vi "Release Queue.vi"(8 "error in (no error)":errorcluster, 11 "Bounded Priority Queue":refnum<class "Bounded Priority Queue.lvclass">) -> (0 "error out":errorcluster, 2 "Remaining Elements":T1[](array[typedef]))   [LabVIEW 2011, in "Bounded Priority Queue.lvclass"]
uses:
  Bounded Priority Queue.lvclass
  Data.ctl
  Bounded Priority Queue.lvclass/Bounded Priority Queue.ctl
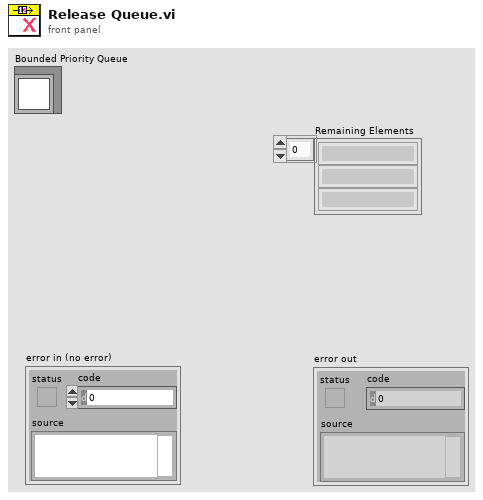
[diagram p1: front panel]
types:
  T1 = typedef "Bounded Priority Queue.lvclass/Data.ctl" = string
  T2 = typedef "Priority Queue.lvclass/DVR Contents.ctl" = cluster{"# Waiting":u32, "Buffers":refnum<queue>[], "How Many Priorities":u32, "Bounding":refnum<queue>}
  T3 = typedef "Priority Queue.lvclass/Data.ctl" = string
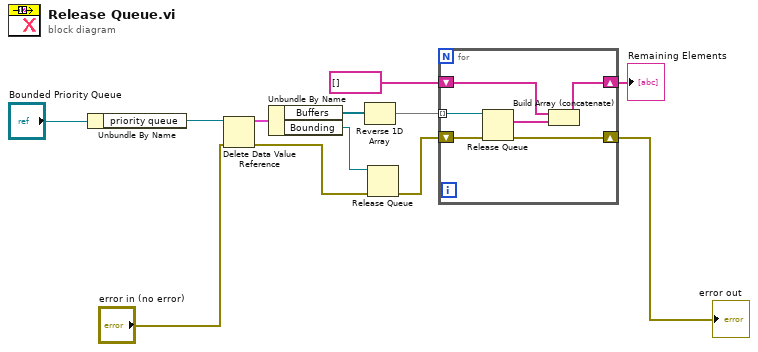
[diagram p0: block diagram]
diagram:
  n1 = Unbundle By Name("Bounded Priority Queue") -> ("priority queue"=w8:refnum<data-value>)
  n2 = Delete Data Value Reference(data value reference=w8, error in="error in (no error)") -> (data value=w11:T2, error out=w2:errorcluster)
  n3 = Unbundle By Name(w11) -> ("Buffers"=w12:refnum<queue>[], "Bounding"=w3:refnum<queue>)
  n4 = Reverse 1D Array(array=w12) -> (reversed array=w6:refnum<queue>[])
  n5 = Release Queue(queue=w3, error in (no error)=w2) -> (error out=w1:errorcluster)  [unwired: 1 in, 2 out]
  n6 = for {
    tunnel: w6 -> [w18] mode=indexing
    shift-right: [w16] -> w5
    shift-left: T1[] [] -> [w15]
    shift-right: [w13] -> w4
    shift-left: w1 -> [w14]
    n7 = Release Queue(queue=w18, error in (no error)=w14) -> (remaining elements=w17:T3[], error out=w13:errorcluster)  [unwired: 1 in, 1 out]
    n8 = Build Array (concatenate)(w15, w17) -> (w16:T3[])
  }
  "error out" <- w4
  "Remaining Elements" <- w5
